vi "delete control from class private data.vi"(8 "error in":errorcluster, 9 "control label":string, 10 "path":path, 11 "project in":refnum<vi>) -> (0 "error out":errorcluster, 3 "project out":refnum<vi>)   [LabVIEW 2014, in "SequencerActionScript.lvclass"]
doc: "NI Tag Bus Module Framework 1.0.2.36\nNI Systems Engineering"
uses:
  SequencerActionScript.lvclass
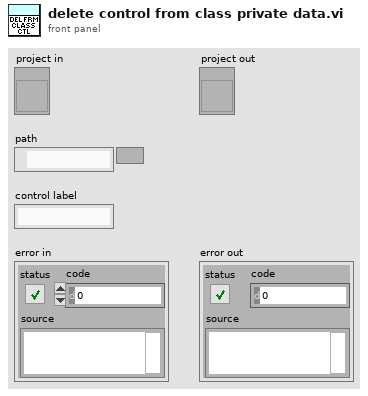
[diagram p1: front panel]
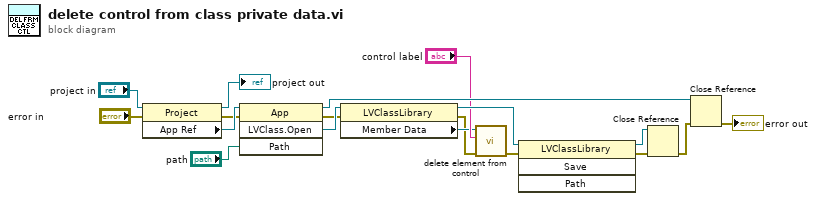
[diagram p0: block diagram]
diagram:
  n1 = property class="Project"(reference="project in", error in="error in") -> (reference out=→"project out":refnum<vi>, error out=w3:errorcluster, "App Ref"=w4:refnum<vi>)
  n2 = invoke class="App" method="LVClass.Open"(reference=w4, error in=w3, "Path"="path") -> (reference out=w14:refnum<vi>, error out=w6:errorcluster, "LVClass.Open"=w7:refnum<vi>)  [unwired: 1 in, 1 out]
  n3 = property class="LVClassLibrary"(reference=w7, error in=w6) -> (reference out=w13:refnum<vi>, error out=w8:errorcluster, "Member Data"=w9:refnum<vi>)
  n4 = call "delete element from control.vi"("error in"=w8, "control label"="control label", "vi in"=w9) -> ("error out"=w15:errorcluster)  [unwired: 8 in]
  n5 = invoke class="LVClassLibrary" method="Save"(reference=w13, error in=w15) -> (reference out=w12:refnum<vi>, error out=w11:errorcluster)  [unwired: 2 in, 2 out]
  n6 = Close Reference(reference=w12, error in (no error)=w11) -> (error out=w16:errorcluster)
  n7 = Close Reference(reference=w14, error in (no error)=w16) -> (error out=→"error out":errorcluster)
